vi "DAQ-PXIe_ReadXML_Config.vi"(8 "error in":errorcluster, 10 "StreamCluster_TypeDef":T5={"DAQ"={"ManagmentRate_Hz"=1000, "StreamRate_Hz"=10, "refDesArray"=[], "StreamRate_ms"=0, "ManagmentRate_ms"=1000}, "Modules"=[]}, 11 "path":path) -> (0 "error out":errorcluster={"status"=TRUE, "code"=0, "source"=""}, 1 "DAQmx Cluster Out":T1 {"ai DAQmx Cluster"."input terminal configuration" items=["Default"=-1, "RSE"=10083, "NRSE"=10078, "Differential"=10106, "Pseudodifferential"=12529]; "bc DAQmx Cluster"."Scaling Information"."electrical units" items=["Volts/Volt"=15896, "mVolts/Volt"=15897]; "bc DAQmx Cluster"."Scaling Information"."physical units" items=["Newtons"=15875, "Pounds"=15876, "kgf"=15877]; "bc DAQmx Cluster"."Bridge Information"."bridge configuration" items=["Full Bridge"=10182, "Half Bridge"=10187, "Quarter Bridge"=10270]; "bc DAQmx Cluster"."Bridge Information"."voltage excitation source" items=["Internal"=10200, "External"=10167]; "tc DAQmx Cluster"."Thermocouple Type" items=["J"=10072, "K"=10073, "N"=10077, "R"=10082, "S"=10085, "T"=10086, "B"=10047, "E"=10055]; "tc DAQmx Cluster"."Units" items=["Deg C"=10143, "Deg F"=10144, "Kelvins"=10325, "Deg R"=10145, "From Custom Scale"=10065]}, 2 "StreamCluster_TypeDef out":T3={"DAQ_Configs"=[], "CTR_Config"={"CTR refDes"="", "CTR IP Addr"="localhost", "Restart"=FALSE}, "Network_Configs"={"Buffer"=1, "ManagmentRate_Hz"=1000, "StreamRate_Hz"=10, "ConnectionHysterisis"=0, "LoggingRate_Hz"=10}, "ConfigXML_Checksum"="210cc09a95e8171523621a6e0fe6cc62ee78011ce952e85bacd084a90afd4457596a89e2a0760488e968f21beda495caaa4ef384b0090342ba5af4eb26a7085d"}, 3 "Calibration Configuration Out":T2)   [LabVIEW 2024]
uses:
  <vilib>/xml/NI_XML.lvlib
  <vilib>/security/Message Digest/API/NI_Message Digest API.lvlib
  Configuration/DAQmx Configuration.ctl
  Configuration/Calibration Configuration.ctl
  <vilib>/xml/Load XML File.vi
  <vilib>/security/Message Digest/API/Instances/File/SHA3-512 File Checksum.vi
  <vilib>/ErrorRing/Error Ring.xnode
  <vilib>/Utility/error.llb/Error Cluster From Error Code.vi
  <vilib>/xml/Close Reference(Node).vi
  Control/streamIO_states.ctl
  Control/StreamCluster_TypeDef.ctl
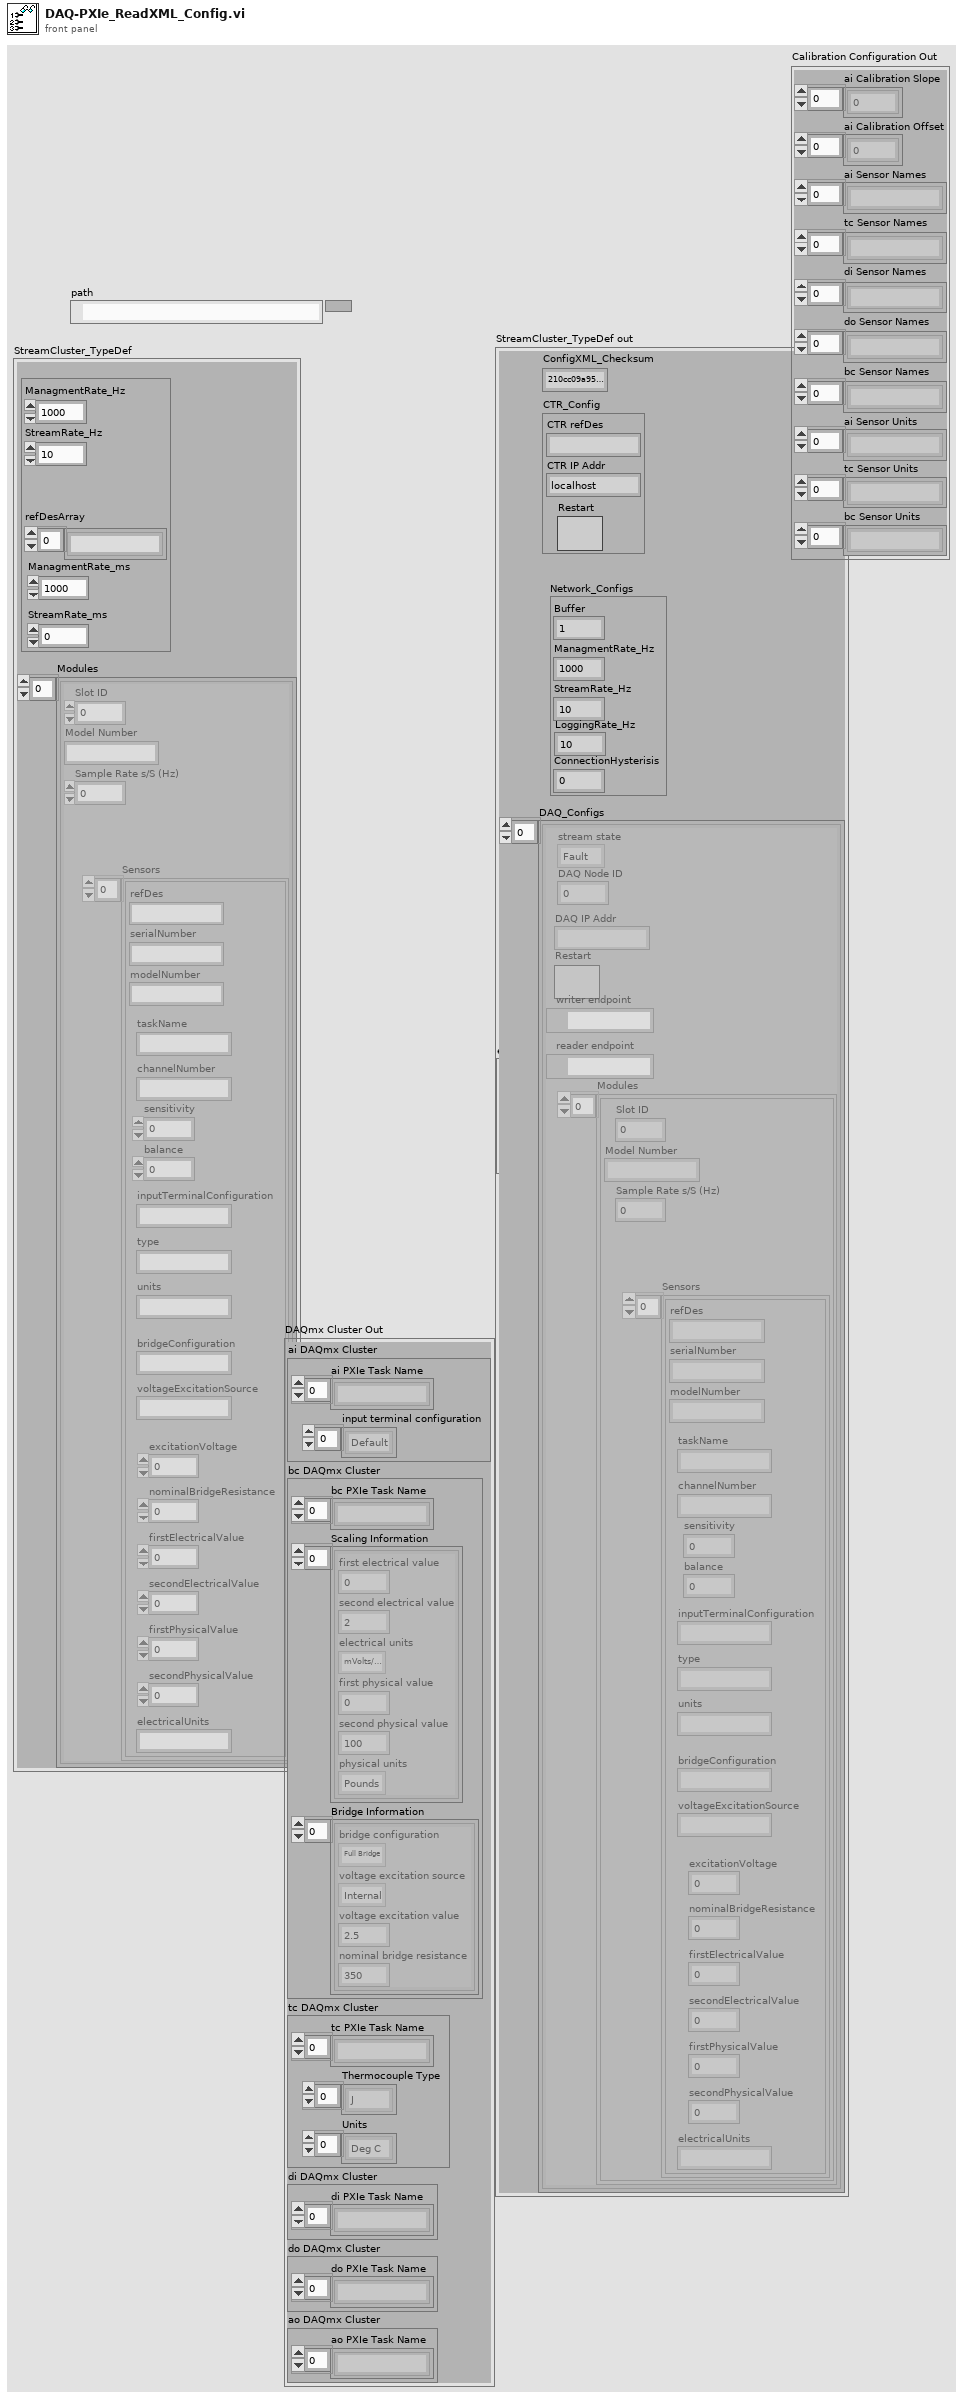
[diagram p1: front panel]
types:
  T1 = typedef "DAQmx Configuration.ctl" = cluster{"ai DAQmx Cluster":cluster{"ai PXIe Task Name":string[], "input terminal configuration":i32[]}, "bc DAQmx Cluster":cluster{"bc PXIe Task Name":string[], "Scaling Information":cluster{"first electrical value":dbl, "second electrical value":dbl, "electrical units":i32, "first physical value":dbl, "second physical value":dbl, "physical units":i32}[], "Bridge Information":cluster{"bridge configuration":i32, "voltage excitation source":i32, "voltage excitation value":dbl, "nominal bridge resistance":dbl}[]}, "tc DAQmx Cluster":cluster{"tc PXIe Task Name":string[], "Thermocouple Type":i32[], "Units":i32[]}, "di DAQmx Cluster":cluster{"di PXIe Task Name":string[]}, "do DAQmx Cluster":cluster{"do PXIe Task Name":string[]}, "ao DAQmx Cluster":cluster{"ao PXIe Task Name":string[]}}
  T2 = typedef "Calibration Configuration.ctl" = cluster{"ai Calibration Slope":dbl[], "ai Calibration Offset":dbl[], "ai Sensor Names ":string[], "tc Sensor Names":string[], "di Sensor Names":string[], "do Sensor Names":string[], "bc Sensor Names":string[], "ai Sensor Units":string[], "tc Sensor Units":string[], "bc Sensor Units":string[]}
  T3 = typedef "StreamCluster_TypeDef.ctl" = cluster{"DAQ_Configs":cluster{"stream state":T4, "DAQ Node ID":i32, "Modules":cluster{"Slot ID":i32, "Model Number":string, "Sample Rate s/S (Hz)":dbl, "Sensors":cluster{"refDes":string, "serialNumber":string, "modelNumber":string, "units":string, "balance":dbl, "sensitivity":dbl, "type":string, "inputTerminalConfiguration":string, "channelNumber":string, "taskName":string, "bridgeConfiguration":string, "excitationVoltage":dbl, "voltageExcitationSource":string, "nominalBridgeResistance":dbl, "firstElectricalValue":dbl, "secondElectricalValue":dbl, "firstPhysicalValue":dbl, "secondPhysicalValue":dbl, "electricalUnits":string}[]}[], "DAQ IP Addr":string, "Restart":bool, "writer endpoint":refnum<k21>, "reader endpoint":refnum<k21>}[], "CTR_Config":cluster{"CTR refDes":string, "CTR IP Addr":string, "Restart":bool}, "Network_Configs":cluster{"Buffer":i32, "ManagmentRate_Hz":i32, "StreamRate_Hz":i32, "ConnectionHysterisis":i32, "LoggingRate_Hz":i32}, "ConfigXML_Checksum":string}
  T4 = typedef "streamIO_states.ctl" = enum16{"Fault", "Initialize", "Stream", "Close"}
  T5 = typedef "StreamCluster_TypeDef.ctl" = cluster{"DAQ":cluster{"ManagmentRate_Hz":i32, "StreamRate_Hz":i32, "refDesArray":string[], "StreamRate_ms":i32, "ManagmentRate_ms":i32}, "Modules":cluster{"Slot ID":i32, "Model Number":string, "Sample Rate s/S (Hz)":dbl, "Sensors":cluster{"refDes":string, "serialNumber":string, "modelNumber":string, "units":string, "balance":dbl, "sensitivity":dbl, "type":string, "inputTerminalConfiguration":string, "channelNumber":string, "taskName":string, "bridgeConfiguration":string, "excitationVoltage":dbl, "voltageExcitationSource":string, "nominalBridgeResistance":dbl, "firstElectricalValue":dbl, "secondElectricalValue":dbl, "firstPhysicalValue":dbl, "secondPhysicalValue":dbl, "electricalUnits":string}[]}[]}
  T6 = typedef "DAQ_channelDefinitions.ctl" = cluster{"refDesDAQ":string, "moduleModel":string, "refDesSensor":string, "channelNumber":string, "modelNumber":string, "serialNumber":string, "Cluster":cluster{"tags":string[], "channels":string[]}}[]
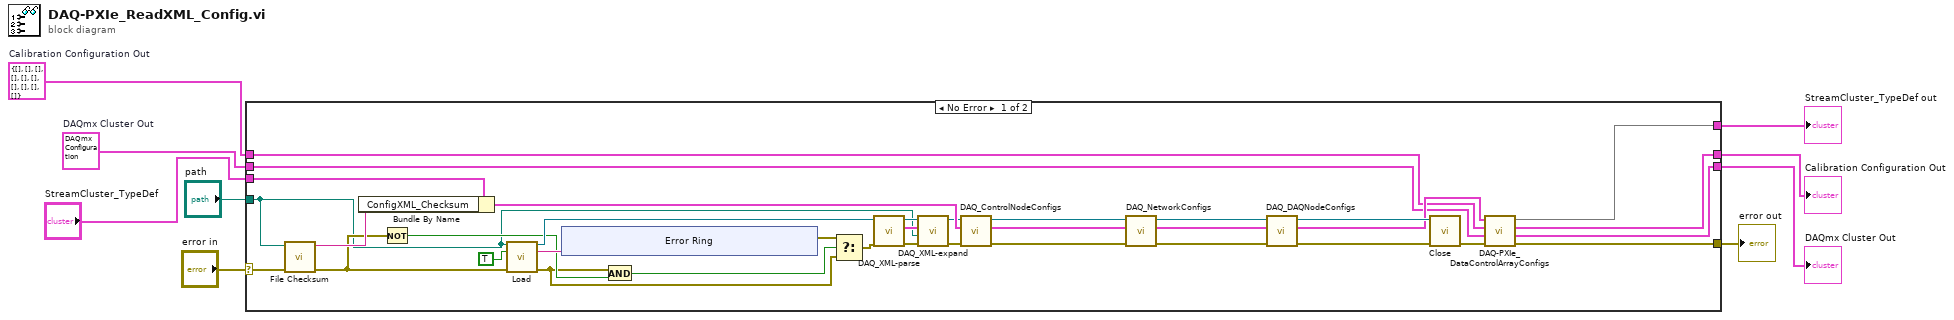
[diagram p0: block diagram]
diagram:
  w2 = T2 {"ai Calibration Slope"=[], "ai Calibration Offset"=[], "ai Sensor Names "=[], "tc Sensor Names"=[], "di Sensor Names"=[], "do Sensor Names"=[], "bc Sensor Names"=[], "ai Sensor Units"=[], "tc Sensor Units"=[], "bc Sensor Units"=[]}  # Calibration Configuration Out
  w1 = T1 {"ai DAQmx Cluster"={"ai PXIe Task Name"=[], "input terminal configuration"=[]}, "bc DAQmx Cluster"={"bc PXIe Task Name"=[], "Scaling Information"=[], "Bridge Information"=[]}, "tc DAQmx Cluster"={"tc PXIe Task Name"=[], "Thermocouple Type"=[], "Units"=[]}, "di DAQmx Cluster"={"di PXIe Task Name"=[]}, "do DAQmx Cluster"={"do PXIe Task Name"=[]}, "ao DAQmx Cluster"={"ao PXIe Task Name"=[]}}  # DAQmx Cluster Out
  n1 = case shown="No Error" "error in" {
    selector: "error in" -> [w44 w55]
    tunnel: [w30 w55] -> w7
    tunnel: "path" -> [w10 _]
    tunnel: "StreamCluster_TypeDef" -> [w40 w54]
    tunnel: [w28 w54] -> w5
    tunnel: [w25 w53] -> w4
    tunnel: [w24 w52] -> w3
    tunnel: w2 -> [w27 w53]
    tunnel: w1 -> [w26 w52]
    frame No Error {
      n2 = call-poly <vilib>:"File Checksum.vi"("error in"=w44, "path"=w10) -> ("error out"=w21:errorcluster, "digest"=w38:string)  [unwired: 8 in]
      n3 = Bundle By Name(cluster=w40, "ConfigXML_Checksum"=w38) -> (w39:T5)
      n4 = Not(x=w21) -> (.not. x?=w20:bool)
      n5 = call-poly <vilib>:"Load.vi"("path to XML document"=w10, "process namespaces (False)"=TRUE, "error in (no error)"=w21) -> ("DOM document out"=w23:refnum<k20>, "parse errors"=w22:string, "error out"=w18:errorcluster)  [unwired: 10 in]
      n6 = xnode "Error Ring"("parameter 0"=w22) -> ("error out"=w17:errorcluster)
      n7 = And(x=w18, y=w20) -> (x .and. y?=w19:bool)
      n8 = Select(t=w17, s=w19, f=w18) -> (s? t:f=w16:errorcluster)
      n9 = call "DAQ_XML-parse.vi"("error in"=w16, "DOM document in"=w23) -> ("error out"=w14:errorcluster, "channel Definitions out"=w11:T6, "DOM document out"=w15:refnum<k20>)  [unwired: 7 in]
      n10 = call "DAQ_XML-expand.vi"("error in"=w14, "XML file path"=w10, "channel Definitions"=w11, "DOM document in"=w15) -> ("error out"=w13:errorcluster, "DOM document out"=w12:refnum<k20>)  [unwired: 6 in]
      n11 = call "DAQ_ControlNodeConfigs.vi"("error in"=w13, "StreamCluster_TypeDef in"=w39, "DOM document in"=w12) -> ("error out"=w41:errorcluster, "StreamCluster_TypeDef out"=w37:T5, "DOM document out"=w42:refnum<k20>)  [unwired: 6 in]
      n12 = call "DAQ_NetworkConfigs.vi"("error in"=w41, "StreamCluster_TypeDef"=w37, "DOM document in"=w42) -> ("error out"=w36:errorcluster, "StreamCluster_TypeDef 2"=w35:T5, "DOM document out"=w34:refnum<k20>)  [unwired: 6 in]
      n13 = call "DAQ_DAQNodeConfigs.vi"("error in"=w36, "StreamCluster_TypeDef in"=w35, "DOM document in"=w34) -> ("error out"=w33:errorcluster, "StreamCluster_TypeDef out"=w29:T5, "DOM document out"=w32:refnum<k20>)  [unwired: 6 in]
      n14 = call-poly <vilib>:"Close.vi"("error in (no error)"=w33, "node"=w32) -> ("error out"=w31:errorcluster)  [unwired: 7 in]
      n15 = call "DAQ-PXIe_DataControlArrayConfigs.vi"("error in"=w31, "DAQmx Cluster In"=w26, "Calibration Configuration In"=w27, "StreamCluster_TypeDef"=w29) -> ("error out"=w30:errorcluster, "DAQmx Cluster Out"=w24:T1, "Calibration Configuration Out"=w25:T2, 3:w28)  [unwired: 4 in]
    }
    frame Error {
    }
  }
  "error out" <- w7
  "StreamCluster_TypeDef out" <- w5
  "Calibration Configuration Out" <- w4
  "DAQmx Cluster Out" <- w3
